vi "Process.vi"(8 "error in":errorcluster, 11 "Example Instrument UI":refnum<class "Instrument UI.Element2.lvclass">) -> (0 "error out":errorcluster, 3 "Example Instrument UI out":refnum<class "Instrument UI.Element2.lvclass">)   [LabVIEW 2019, in "Instrument UI.Element2.lvclass"]
doc: "---------------------------------------------------------------\nJKI State Machine Objects™\nhttp://jki.net/state-machine-objects/\nCopyright (C) 2005-2015, JKI <info@jki.net>\nALL RIGHTS RESERVEDJKI State Machine Objects (SMO) 1.0.0.5\nJKI - JKI\nCopyright (c) 2016, JKI"
uses:
  Instrument UI.Element2.lvclass
  C:/Program Files (x86)/National Instruments/LabVIEW 2019/vi.lib/JKI/JKI SMO/SMO/SMO.lvclass
  C:/Program Files (x86)/National Instruments/LabVIEW 2019/user.lib/LevyLab/Instrument Framework/SMOs/Instrument UI/Instrument UI.lvclass
  C:/Program Files (x86)/National Instruments/LabVIEW 2019/vi.lib/JKI/JKI SMO/SMO.UI/SMO.UI.lvclass
  Instrument.Element2/Typedefs/Instrument.Element2.getAll--Cluster.ctl
  Instrument.Element2/Instrument.Element2.lvclass
  C:/Program Files (x86)/National Instruments/LabVIEW 2019/user.lib/LevyLab/Instrument Framework/SMOs/Instrument/Instrument.lvclass
  Instrument UI.Element2.UI--Cluster.ctl
  Instrument.Element2/Typedefs/Instrument.Element2.Configuration--Cluster.ctl
  <userlib>/LevyLab/Instrument Framework/SMOs/Configuration/Configuration.lvclass
  <userlib>/LevyLab/Instrument Framework/SMOs/Instrument UI/Instrument UI.lvclass/Instrument UI.ctl
  <vilib>/JKI/JKI SMO/SMO/SMO.lvclass/SMO.ctl
  <userlib>/LevyLab/Instrument Framework/SMOs/Instrument/Instrument.lvclass/Instrument.ctl
  Instrument.Element2/Typedefs/Instrument.Element2.Commands--Enum.ctl
  614f1787-3484-4d72-b522-1f8c221dac07.vi
  812ceb25-51ea-4cc0-8aed-c299bc5e652a.vi
  5dc85c1f-8602-43a5-ace5-4d37edcece4b.vi
  199af190-1d6b-4486-8e47-a22270e27068.vi
  f46c0021-6761-4a3c-b250-c526aef0bf8a.vi
  a4c54d18-a951-4ce5-af52-fd32c219282c.vi
  508c6769-fd37-4c88-a163-d37e27e9b26a.vi
  d8b42418-d514-49a9-b82b-7ff31fc1bdce.vi
  4297835d-582f-4ffd-a274-1469935fba4e.vi
  9a5046e7-2a90-4c6a-9e24-f775917da756.vi
  064e3a37-d4cf-416d-9c97-81a00de9d50c.vi
  <vilib>/JKI/JKI SMO/SMO/Private/ReftoDVR--SMO.vi
  614f1787-3484-4d72-b522-1f8c221dac07.vi/8473158c-15b0-4583-96f4-657a0a8663aa.vi
  812ceb25-51ea-4cc0-8aed-c299bc5e652a.vi/b3a63406-e986-4e92-9c3b-61d3b3f5e845.vi
  <userlib>/LevyLab/Instrument Framework/SMOs/Instrument/API/Send and Receive.vi
  5dc85c1f-8602-43a5-ace5-4d37edcece4b.vi/c2ea8b73-9e98-4876-b80f-f9b76f4e6007.vi
  199af190-1d6b-4486-8e47-a22270e27068.vi/885cf8f8-053e-4c02-a193-c26a5fc5fd2e.vi
  f46c0021-6761-4a3c-b250-c526aef0bf8a.vi/d39bdf40-357d-4b84-b6e1-0fa9a47eb352.vi
  a4c54d18-a951-4ce5-af52-fd32c219282c.vi/e6982fbf-8c58-4b4e-8d6c-ef964828a5ea.vi
  508c6769-fd37-4c88-a163-d37e27e9b26a.vi/c2cd9c33-c0f3-4ea8-8363-db61e99eb68f.vi
  d8b42418-d514-49a9-b82b-7ff31fc1bdce.vi/7908e09d-14a4-4f19-b705-d41f2a7bdd7f.vi
  4297835d-582f-4ffd-a274-1469935fba4e.vi/ae23a806-acf6-4b68-963a-90a4cd4bdf43.vi
  9a5046e7-2a90-4c6a-9e24-f775917da756.vi/aa9366ea-5b79-4087-9b0d-90153f2fc7d9.vi
  064e3a37-d4cf-416d-9c97-81a00de9d50c.vi/3b377202-371f-4596-b702-b3c926413c9d.vi
  614f1787-3484-4d72-b522-1f8c221dac07.vi/8473158c-15b0-4583-96f4-657a0a8663aa.vi/a83233ea-3f32-419c-97c8-4d037e5cf615.vi
  812ceb25-51ea-4cc0-8aed-c299bc5e652a.vi/b3a63406-e986-4e92-9c3b-61d3b3f5e845.vi/6ae25757-18c0-4edf-8ec6-5ee7498e42bc.vi
  812ceb25-51ea-4cc0-8aed-c299bc5e652a.vi/b3a63406-e986-4e92-9c3b-61d3b3f5e845.vi/ba664fe4-fbf7-4d22-b628-f2801aca82a6.vi
  5dc85c1f-8602-43a5-ace5-4d37edcece4b.vi/c2ea8b73-9e98-4876-b80f-f9b76f4e6007.vi/1e7106c2-e63d-4954-be79-ade3d086157d.vi
  5dc85c1f-8602-43a5-ace5-4d37edcece4b.vi/c2ea8b73-9e98-4876-b80f-f9b76f4e6007.vi/5273b4ab-85e4-43b8-966e-2f27bfd0b167.vi
  199af190-1d6b-4486-8e47-a22270e27068.vi/885cf8f8-053e-4c02-a193-c26a5fc5fd2e.vi/98bda066-dba2-44b6-a77b-658504ed82f7.vi
  199af190-1d6b-4486-8e47-a22270e27068.vi/885cf8f8-053e-4c02-a193-c26a5fc5fd2e.vi/85f2e53d-7bfa-45b4-936c-816543ada8b5.vi
  f46c0021-6761-4a3c-b250-c526aef0bf8a.vi/d39bdf40-357d-4b84-b6e1-0fa9a47eb352.vi/fff4bc55-b81b-4902-9052-ccea61a7805f.vi
  f46c0021-6761-4a3c-b250-c526aef0bf8a.vi/d39bdf40-357d-4b84-b6e1-0fa9a47eb352.vi/8e797443-0d66-4240-84e1-5cfe0d1267f8.vi
  a4c54d18-a951-4ce5-af52-fd32c219282c.vi/e6982fbf-8c58-4b4e-8d6c-ef964828a5ea.vi/d1cd9f94-2750-44a9-b431-0a9c43ba5784.vi
  a4c54d18-a951-4ce5-af52-fd32c219282c.vi/e6982fbf-8c58-4b4e-8d6c-ef964828a5ea.vi/7fd59099-3350-4db8-8eec-f4e447bc4942.vi
  508c6769-fd37-4c88-a163-d37e27e9b26a.vi/c2cd9c33-c0f3-4ea8-8363-db61e99eb68f.vi/e3fa67e6-a539-4712-b44b-6125dcbb05d4.vi
  508c6769-fd37-4c88-a163-d37e27e9b26a.vi/c2cd9c33-c0f3-4ea8-8363-db61e99eb68f.vi/023fab8a-09d3-4eb7-ae02-fd4ece76aac4.vi
  d8b42418-d514-49a9-b82b-7ff31fc1bdce.vi/7908e09d-14a4-4f19-b705-d41f2a7bdd7f.vi/0e3d71bf-4189-4105-849b-527ecaac9cd6.vi
  d8b42418-d514-49a9-b82b-7ff31fc1bdce.vi/7908e09d-14a4-4f19-b705-d41f2a7bdd7f.vi/ea41837a-8cf8-405a-9125-7913f32814bd.vi
  4297835d-582f-4ffd-a274-1469935fba4e.vi/ae23a806-acf6-4b68-963a-90a4cd4bdf43.vi/9f397512-bf51-4fde-81a7-7db753787438.vi
  4297835d-582f-4ffd-a274-1469935fba4e.vi/ae23a806-acf6-4b68-963a-90a4cd4bdf43.vi/dd848b74-03c7-4bc3-8844-5b3e47300b5e.vi
  9a5046e7-2a90-4c6a-9e24-f775917da756.vi/aa9366ea-5b79-4087-9b0d-90153f2fc7d9.vi/42cffef1-50ff-4d5f-87eb-c31c2d9921ce.vi
  9a5046e7-2a90-4c6a-9e24-f775917da756.vi/aa9366ea-5b79-4087-9b0d-90153f2fc7d9.vi/f97c7ae1-12fc-4289-a497-f57069b3a3b7.vi
  064e3a37-d4cf-416d-9c97-81a00de9d50c.vi/3b377202-371f-4596-b702-b3c926413c9d.vi/9a630cf9-65e1-4d6a-a759-0b0e5b61d144.vi
  614f1787-3484-4d72-b522-1f8c221dac07.vi/8473158c-15b0-4583-96f4-657a0a8663aa.vi/a83233ea-3f32-419c-97c8-4d037e5cf615.vi/7e6555d9-0260-4203-9cda-f5732bbb5bfe.vi
  614f1787-3484-4d72-b522-1f8c221dac07.vi/8473158c-15b0-4583-96f4-657a0a8663aa.vi/a83233ea-3f32-419c-97c8-4d037e5cf615.vi/e950cb7d-6eaf-4b82-ab84-ba08af2cf0bb.vi
  064e3a37-d4cf-416d-9c97-81a00de9d50c.vi/3b377202-371f-4596-b702-b3c926413c9d.vi/9a630cf9-65e1-4d6a-a759-0b0e5b61d144.vi/9bda2bf0-22a8-471b-9ceb-dc726eacd9f3.vi
  064e3a37-d4cf-416d-9c97-81a00de9d50c.vi/3b377202-371f-4596-b702-b3c926413c9d.vi/9a630cf9-65e1-4d6a-a759-0b0e5b61d144.vi/6c670a7e-983d-46cc-b509-b9c25e863d4c.vi
  <userlib>/LevyLab/Instrument Framework/SMOs/Instrument/API/Enum to String.vi
  <userlib>/LevyLab/Instrument Framework/SMOs/RemoteControl/API/Send and Receive.vi
  <vilib>/Utility/Data Type/Get Type Information.vi
  <vilib>/JDP Science/JSONtext/JSON text to Variant.vi
  <userlib>/LevyLab/Instrument Framework/SMOs/Instrument/Instrument.lvclass
  <vilib>/JDP Science/JSONtext/LVClass Serializer/JSONtext LVClass Serializer.lvclass
  <userlib>/LevyLab/Instrument Framework/SMOs/Instrument UI/Instrument UI.lvclass
  <vilib>/JKI/JKI SMO/SMO/SMO.lvclass
  <vilib>/JKI/JKI SMO/SMO.UI/SMO.UI.lvclass
panel:
  out "Diode Current (A)":dbl
  out "Temperature (C)":dbl
  out "Error":bool
  out "Shutter":bool
  out "Laser":bool
  in  "Send Custom":bool
  in  "CustomString":string
  in  "Clear Errors":bool
  in  "Update Time":bool
  in  "Clear Shutdown":bool
  in  "Clear Wakeup":bool
  in  "Set Shutdown":bool
  in  "Shutdown Time":timestamp
  in  "Stop":bool
  in  "Start":bool
  out "Pump Power (W)":dbl
  in  "Wakeup Time":timestamp
  out "Status":string
  in  "Parameter 2":string
  out "Numeric":u32
  in  "Set Wakeup":bool
  in  "Parameter":dbl
  in  "Exit":bool
  # "Element 2 Monitor"
  # "SMO UI Template"
  # "For instructions on how to use the JKI State Machine Objects, examples and video tutorials, visit:\nhttp://jki.net/state-machine-objects/\n\nJKI State Machine Objects™\nhttp://jki.net/state-machine-objects/\nCopyright (C) 2005-2015, JKI <info@jki.net>\nALL RIGHTS RESERVED"
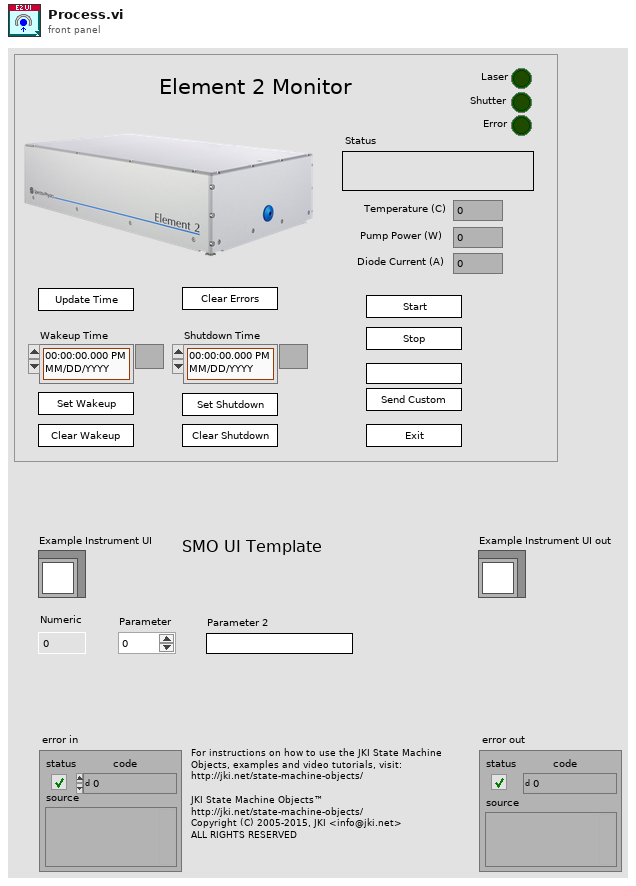
[diagram p1: front panel]
types:
  T1 = enum32{"invalid app kind", "Development System", "Run Time System", "Student Edition", "Embedded LabVIEW", "Evaluation", "Custom"}
  T2 = enum32{"Invalid", "Standard", "Closed", "Hidden", "Minimized", "Maximized"}
  T3 = typedef "Instrument.Element2.lvclass/Instrument.Element2.Commands--Enum.ctl" = enum16{"Start", "Stop", "Set Wakeup", "Clear Wakeup", "Set Shutdown", "Clear Shutdown", "Clear Errors", "Update Time", "Send Custom"}
  T4 = typedef "Instrument.Element2.lvclass/Instrument.Element2.Configuration--Cluster.ctl" = cluster{"Example Setting 1":dbl}
  T5 = typedef "Instrument.Element2.lvclass/Instrument.Element2.getAll--Cluster.ctl" = cluster{"Pump Power":dbl, "Laser Status":string, "Startup/Shutdown Status":string, "Diode Current Set":dbl, "Diode Current Actual":dbl, "Temp: Pump Chassis":dbl, "Temp: Pump PCB":dbl, "Temp: Pump Tower":dbl, "Temp: Pump Diodes":dbl, "Temp: Control Unit":dbl, "Temp: Laser Head Pos 1":dbl, "Temp: Laser Head Pos 2":dbl}
  T6 = typedef "Instrument UI.Element2.lvclass/Instrument UI.Element2.UI--Cluster.ctl" = cluster{"Parameter":dbl, "Parameter 2":string}
  T7 = cluster{"Core":cluster{"Current VI Reference":refnum<vi>, "Close Panel on Exit?":bool, "error":errorcluster}, "Instrument UI":refnum<class "Instrument UI.Element2.lvclass">, "Instrument":refnum<class "Instrument.Element2.lvclass">, "Configuration":refnum<class "Configuration.lvclass">, "Config Cluster":T4, "getAll":T5, "UI Cluster":T6}
  T8 = cluster{"Current VI Reference":refnum<vi>, "Close Panel on Exit?":bool, "error":errorcluster}
  T9 = typedef "SMO.lvclass/Protected Events.ctl" = cluster{"StopProcesses":refnum<user-event>, "AbortProcesses":refnum<user-event>, "Config Changed":refnum<user-event>, "Dependency":refnum<user-event>}
  T10 = typedef "Instrument.lvclass/PublicEvents--Cluster.ctl" = cluster{"MessageFromProcess":refnum<user-event>}
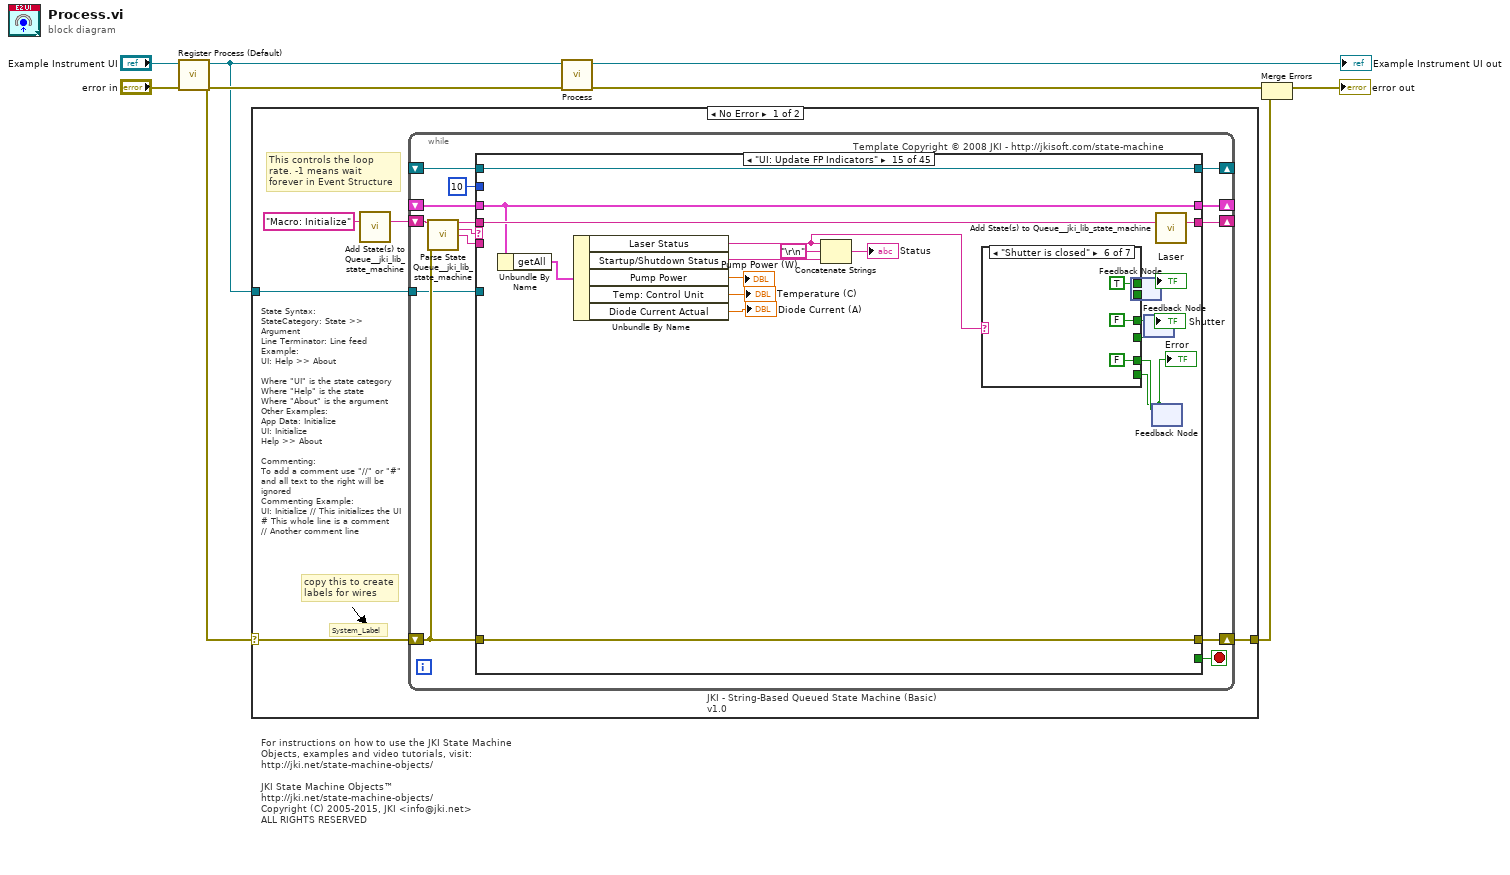
[diagram p0: block diagram]
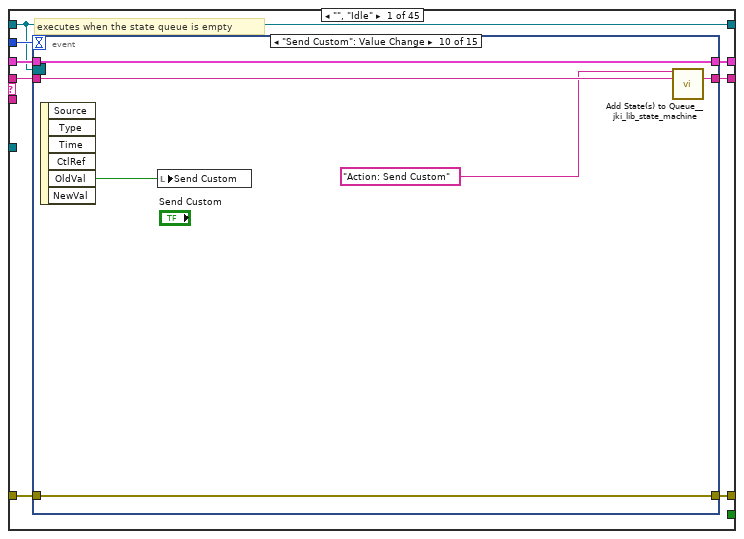
[diagram p2: hidden frame]
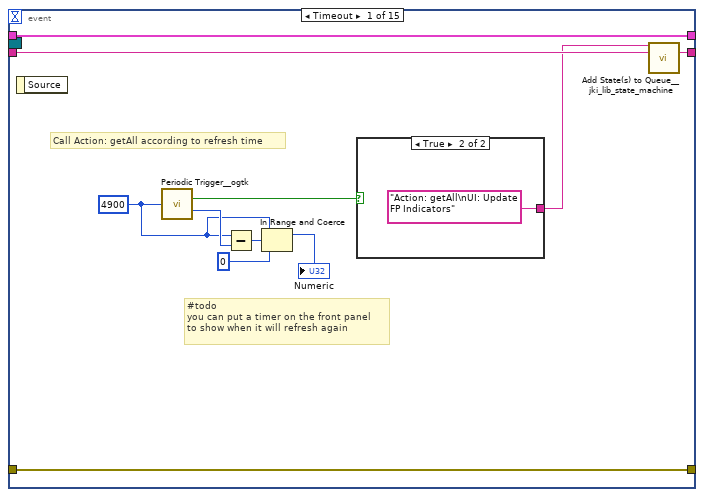
[diagram p3: hidden frame]
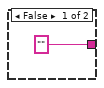
[diagram p4: hidden frame]
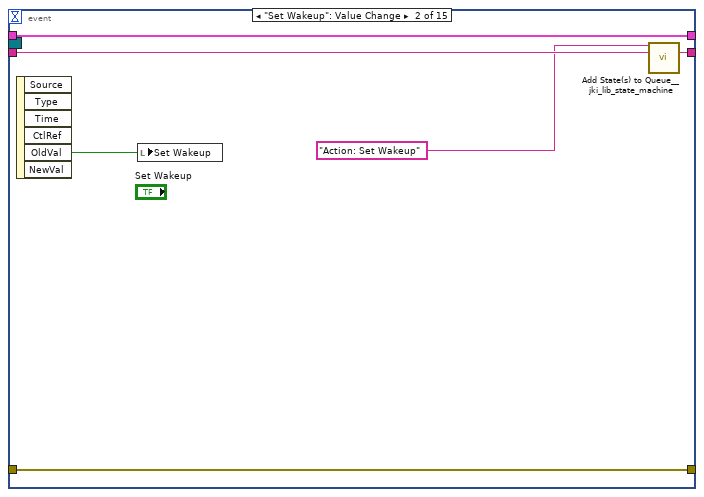
[diagram p5: hidden frame]
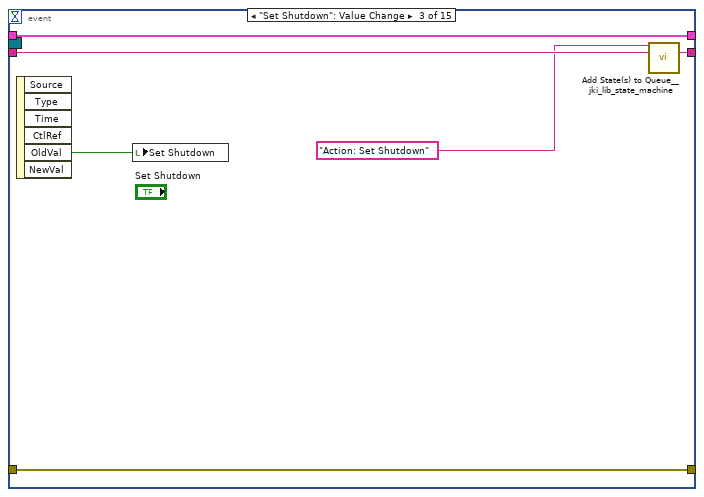
[diagram p6: hidden frame]
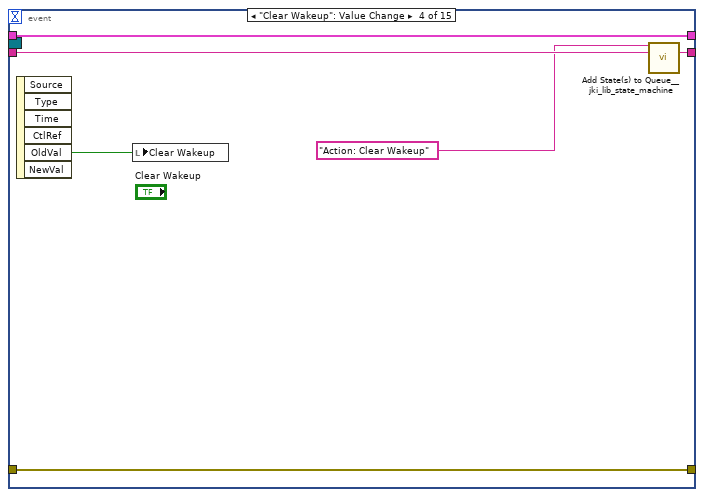
[diagram p7: hidden frame]
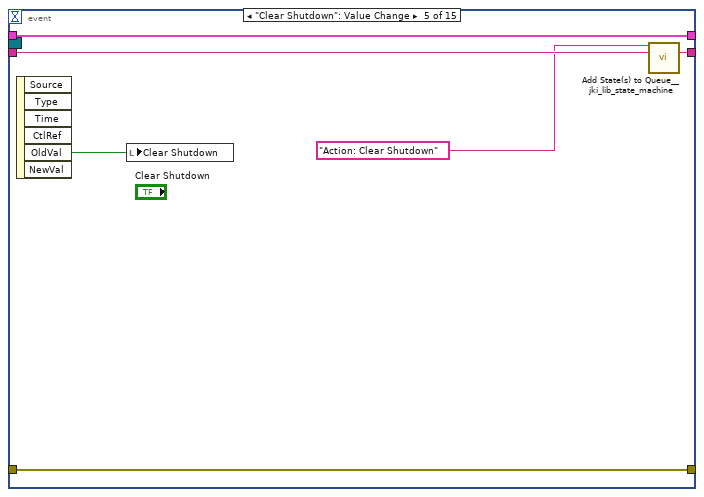
[diagram p8: hidden frame]
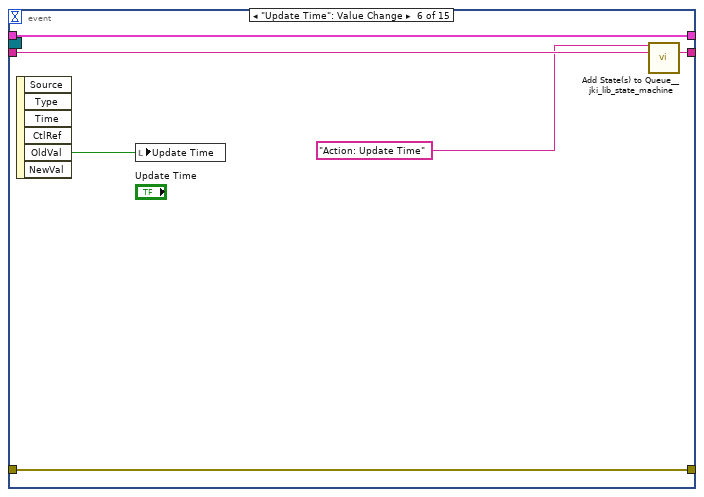
[diagram p9: hidden frame]
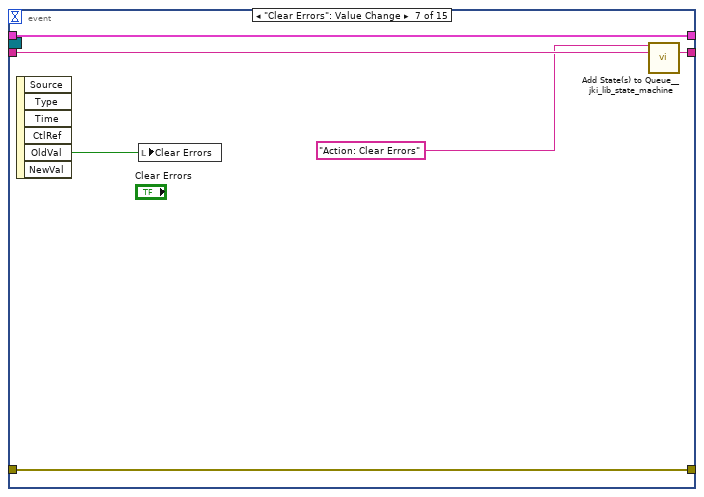
[diagram p10: hidden frame]
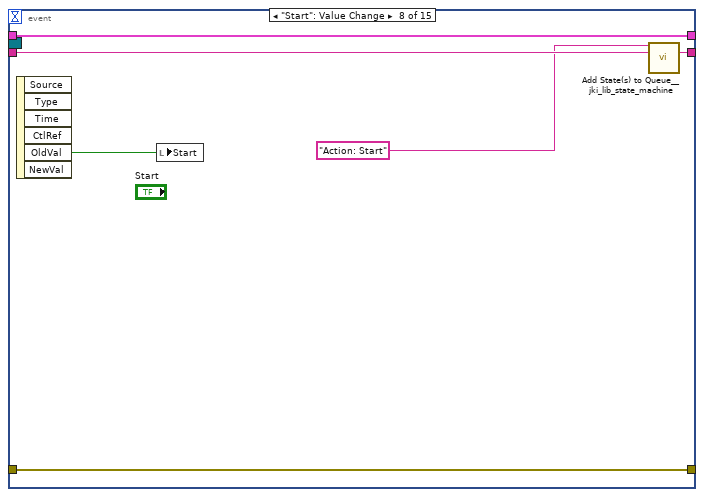
[diagram p11: hidden frame]
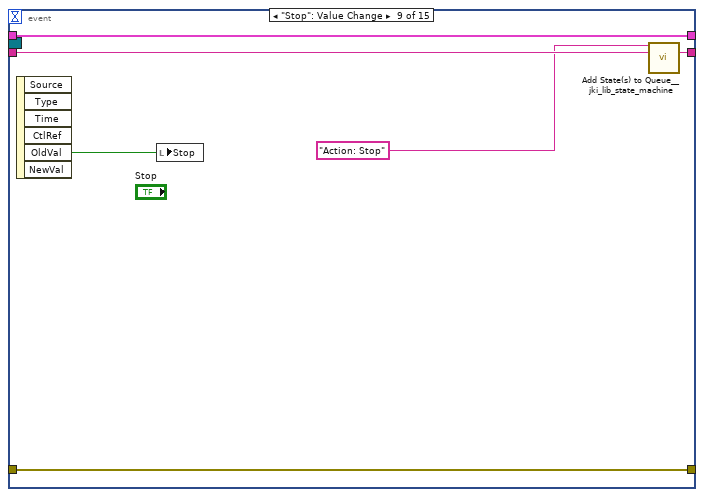
[diagram p12: hidden frame]
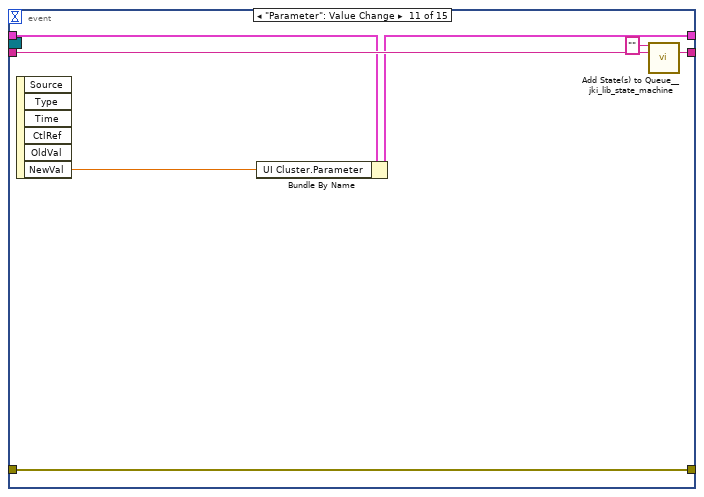
[diagram p13: hidden frame]
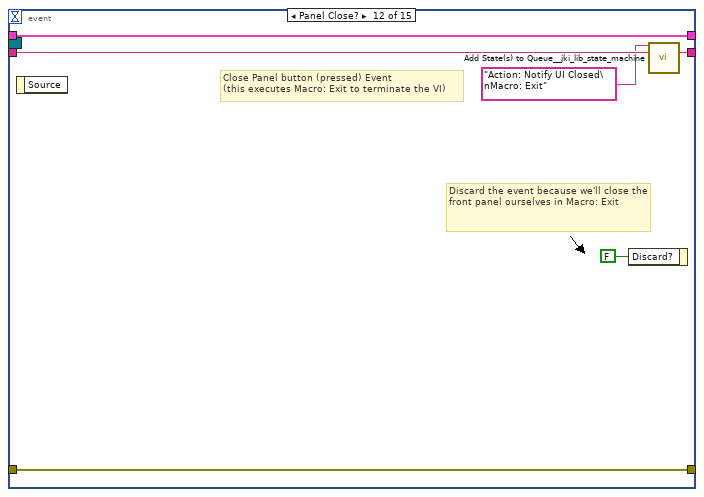
[diagram p14: hidden frame]
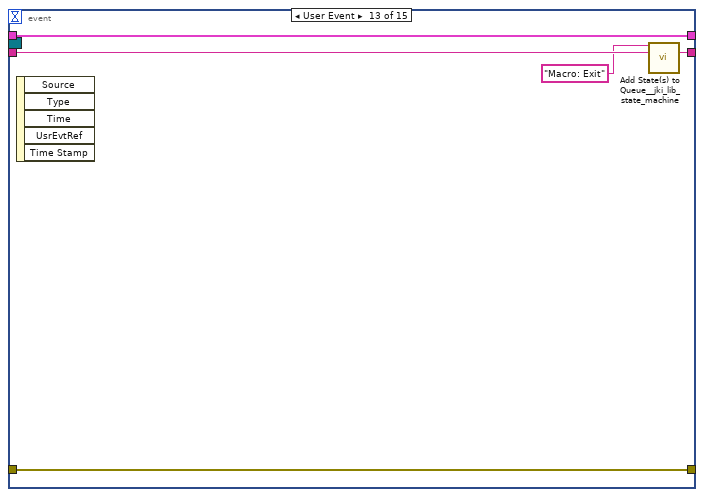
[diagram p15: hidden frame]
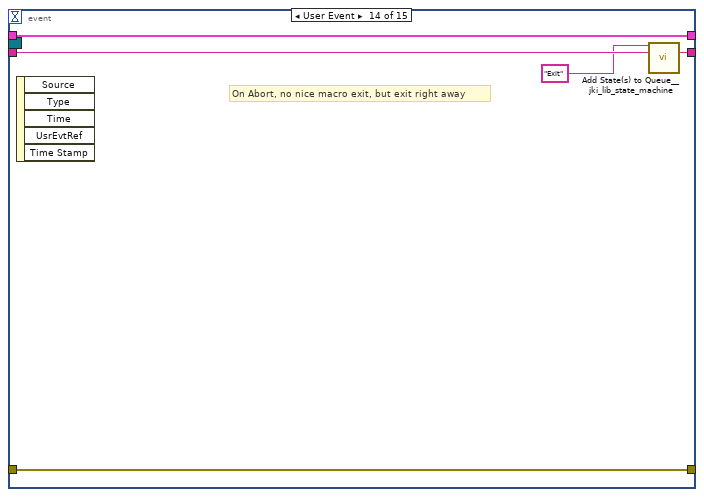
[diagram p16: hidden frame]
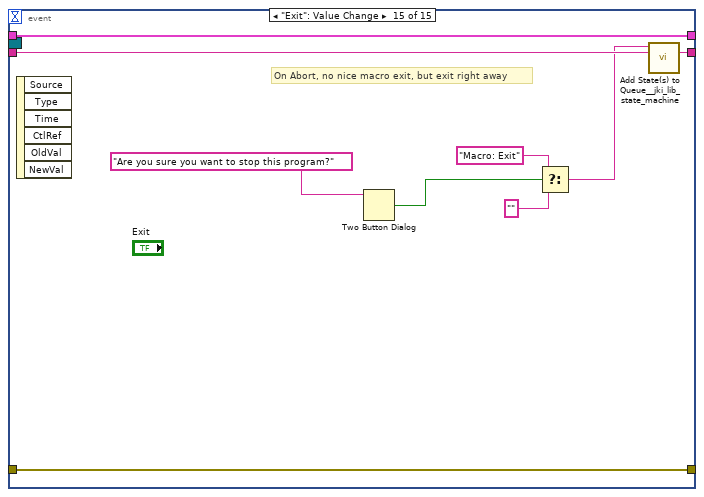
[diagram p17: hidden frame]
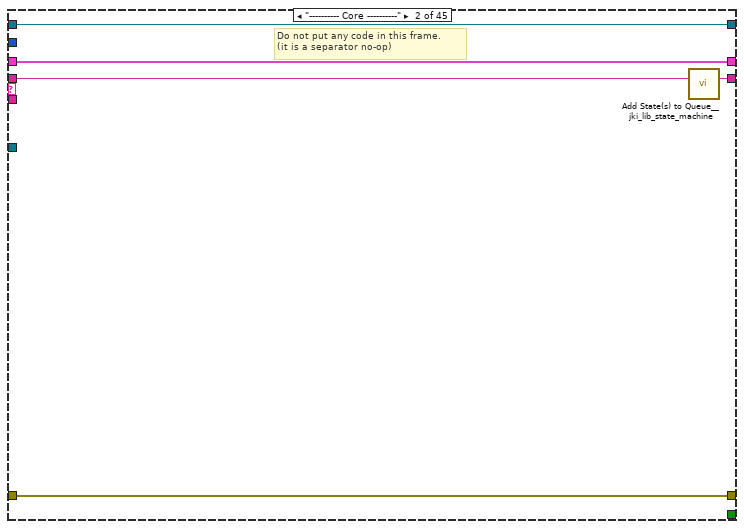
[diagram p18: hidden frame]
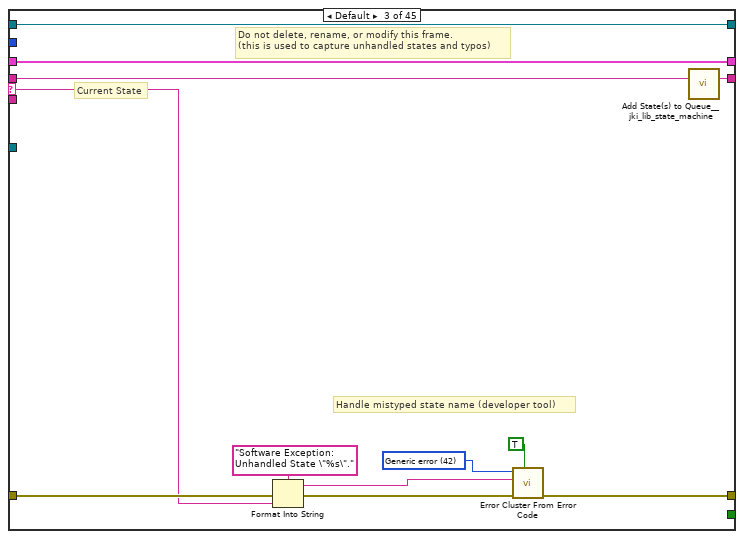
[diagram p19: hidden frame]
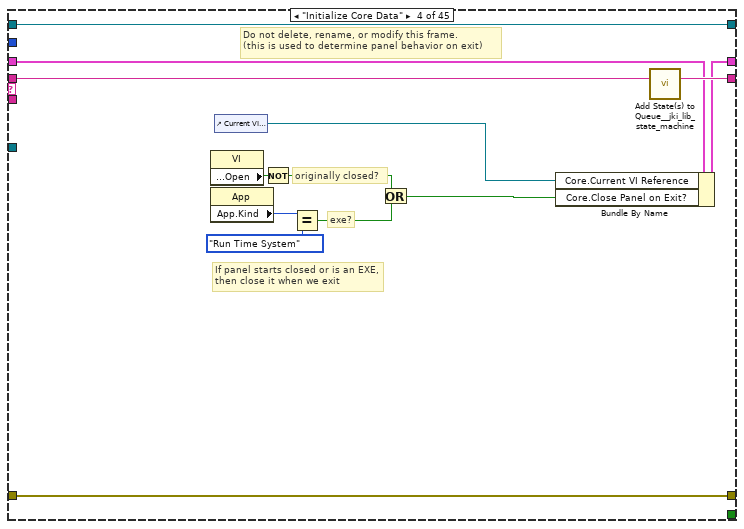
[diagram p20: hidden frame]
diagram:
  # "For instructions on how to use the JKI State Machine Objects, examples and video tutorials, visit:\nhttp://jki.net/state-machine-objects/\n\nJKI State Machine Objects™\nhttp://jki.net/state-machine-objects/\nCopyright (C) 2005-2015, JKI <info@jki.net>\nALL RIGHTS RESERVED"
  n1 = call <vilib>:"Register Process (Default).vi"("error in (no error)"="error in", "SMO"="Example Instrument UI") -> ("error out"=w5:errorcluster, "SelfRef"=w4:refnum<class "Instrument UI.Element2.lvclass">)  [unwired: 8 in]
  n2 = case shown="No Error" w5 {
    selector: w5 -> [w10 w603]
    tunnel: w4 -> [w11 _]
    tunnel: [w9 w603] -> w1
    frame No Error {
      # "State Syntax:\nStateCategory: State >> Argument\nLine Terminator: Line feed\nExample:\nUI: Help >> About\n\nWhere \"UI\" is the state category\nWhere \"Help\" is the state\nWhere \"About\" is the argument\nOther Examples:\nApp Data: Initialize\nUI: Initialize\nHelp >> About\n\nCommenting:\nTo add a comment use \"//\" or \"#\" and all text to the right will be ignored\nCommenting Example:\nUI: Initialize // This initializes the UI\n# This whole line is a comment\n// Another comment line"
      # "copy this to create labels for wires"
      # "This controls the loop rate. -1 means wait forever in Event Structure"
      # "System_Label"
      n3 = call <vilib>:"Add State(s) to Queue__jki_lib_state_machine.vi"("State(s) in (\"\")"="Macro: Initialize") -> ("States Out"=w13:string)  [unwired: 14 in]
      n4 = while "JKI - String-Based Queued State Machine (Basic) v1.0" {
        shift-right: [w20] -> _
        shift-left: _ -> [w19]
        shift-right: [w23] -> w9
        shift-left: w10 -> [w17]
        shift-right: [w22] -> _
        shift-left: w13 -> [w24]
        tunnel: w11 -> [w16]
        shift-right: [w15] -> _
        shift-left: _ -> [w14]
        stop <- w21 stop-if-true
        # "Template Copyright © 2008 JKI - http://jkisoft.com/state-machine"
        n5 = call <vilib>:"Parse State Queue__jki_lib_state_machine.vi"("State Queue"=w24, "Error In (no error)"=w17) -> ("Remaining States"=w26:string, "Current State"=w27:string, "Arguments"=w25:string)  [unwired: 11 in]
        n6 = case shown="\"UI: Update FP Indicators\"" w27 {
          selector: w27 -> [_ _ w141 _ _ _ _ _ _ _ _ _ _ _ _ _ _ _ _ _ _ _ _ _ _ _ _ _ _ _ _ _ _ _ _ _ _ _ _ _ _ _ _ _ _]
          tunnel: w26 -> [w35 w139 w145 w164 w178 w184 w189 w209 w217 w222 w229 w234 w241 w248 w267 w295 w311 w343 w352 w358 w364 w379 w384 w395 w402 w407 w420 w426 w431 w443 w451 w463 w470 w477 w489 w501 w513 w524 w535 w546 w557 w568 w579 w591 w602]
          tunnel: w25 -> [_ _ _ _ _ _ _ _ _ _ _ _ _ _ _ w289 w305 _ _ _ _ _ _ _ _ _ _ _ _ _ _ _ _ _ _ _ _ _ _ _ _ _ _ _ _]
          tunnel: w19 -> [w33 w136 w143 w155 w167 w180 w186 _ w213 w218 w223 w231 w239 w244 w262 w293 w307 w340 w348 w355 w361 w366 w381 w392 w397 w404 w418 w424 w428 w434 w448 w454 w466 w471 w481 w496 w508 w519 w530 w541 w552 w563 w574 w586 w594]
          tunnel: [w32 w137 w147 w161 w169 w179 w187 w191 w215 w220 w225 w232 w236 w246 w263 w290 w308 w341 w350 w356 w362 w377 w382 w386 w398 w405 w413 w421 w429 w438 w446 w455 w467 w472 w486 w492 w504 w515 w526 w537 w548 w559 w570 w582 w599] -> w23
          tunnel: w17 -> [w31 w137 w146 w161 w174 _ w187 w206 w215 w220 w226 w232 w237 w246 w263 w291 w309 w341 w350 w356 w362 w377 w382 w387 w399 w405 w415 w422 w429 w436 w444 w456 w467 w473 w482 w493 w505 w516 w527 w538 w549 w560 w571 w583 w595]
          tunnel: [w34 w138 w144 w163 w177 w183 w188 w208 w216 w221 w228 w233 w240 w247 w266 w294 w310 w342 w351 w357 w363 w378 w383 w394 w401 w406 w419 w425 w430 w442 w450 w462 w469 w476 w488 w500 w512 w523 w534 w545 w556 w567 w578 w590 w601] -> w22
          tunnel: [_ _ _ _ _ TRUE _ _ _ _ _ _ _ _ _ _ _ _ _ _ _ _ _ _ _ _ _ _ _ _ _ _ _ _ _ _ _ _ _ _ _ _ _ _ _] -> w21
          tunnel: [w30 w136 w143 w162 w166 w180 w186 w207 w212 w218 w223 w231 w239 w244 w262 w293 w307 w340 w348 w355 w361 w366 w381 w392 w397 w404 w418 w424 w428 w440 w448 w452 w465 w471 w483 w497 w509 w520 w531 w542 w553 w564 w575 w587 w596] -> w20
          tunnel: 10 ("Timeout") -> [w29 _ _ _ _ _ _ _ _ _ _ _ _ _ _ _ _ _ _ _ _ _ _ _ _ _ _ _ _ _ _ _ _ _ _ _ _ _ _ _ _ _ _ _ _]
          tunnel: w16 -> [_ _ _ _ _ _ _ w204 _ _ _ _ _ _ _ _ _ _ _ _ _ _ _ _ _ _ _ _ _ _ _ _ _ _ _ _ _ _ _ _ _ _ _ _ _]
          tunnel: [w28 w135 w140 w152 w176 w181 w185 w203 w214 w219 w224 w230 w238 w245 w265 w292 w304 w339 w349 w354 w360 w371 w380 w393 w400 w403 w417 w423 w427 w441 w449 w461 w468 w475 w487 w499 w511 w522 w533 w544 w555 w566 w577 w589 w600] -> w15
          tunnel: w14 -> [w28 w135 w140 w152 w176 w181 w185 w203 w214 w219 w224 w230 w238 w245 w265 w292 w304 w339 w349 w354 w360 w371 w380 w393 w400 w403 _ w423 w427 w441 w449 w461 w468 w475 w487 w499 w511 w522 w533 w544 w555 w566 w577 w589 w600]
          frame "", "Idle" {
            # "executes when the state queue is empty"
            n7 = event shown="[9] \"Send Custom\": Value Change" {
              selector: w28 -> [_ _ _ _ _ _ _ _ _ _ _ _ _ _ _]
              dyn-events: _ -> [_ _ _ _ _ _ _ _ _ _ _ _ _ _ _]
              timeout: w29 -> [_ _ _ _ _ _ _ _ _ _ _ _ _ _ _]
              tunnel: w35 -> [w46 w54 w60 w66 w72 w78 w84 w90 w96 w102 w109 w115 w120 w125 w134]
              tunnel: [w45 w53 w59 w65 w71 w77 w83 w89 w95 w101 w108 w114 w119 w124 w133] -> w34
              tunnel: w33 -> [w43 w51 w57 w63 w69 w75 w81 w87 w93 w99 w105 w111 w117 w122 w131]
              tunnel: [w44 w52 w58 w64 w70 w76 w82 w88 w94 w100 w107 w110 w118 w123 w132] -> w32
              tunnel: w31 -> [w44 w52 w58 w64 w70 w76 w82 w88 w94 w100 w107 w110 w118 w123 w132]
              tunnel: [w43 w51 w57 w63 w69 w75 w81 w87 w93 w99 w104 w111 w117 w122 w131] -> w30
              event Timeout {
                w37 = u32 4900 ("time (ms)")
                # "#todo\nyou can put a timer on the front panel\nto show when it will refresh again"
                # "Call Action: getAll according to refresh time"
                n8 = event-data() -> ()  [unwired: 1 in, 1 out]
                n9 = call <userlib>:"Periodic Trigger__ogtk.vi"("time (ms)"=w37) -> ("Triggered"=w41:bool, "timer value"=w40:u32)  [unwired: 12 in, 1 out]
                n10 = Subtract(x=w37, y=w40) -> (x-y=w39:u32)
                n11 = In Range and Coerce(upper limit=w37, x=w39, lower limit=u32 0) -> (coerced(x)=→"Numeric":u32)  [unwired: 1 out]
                n12 = case shown="True" w41 {
                  tunnel: ["" ("State(s) in Front (\"\")") "Action: getAll\nUI: Update FP Indicators" ("State(s) in Front (\"\")")] -> w42
                  frame False {
                  }
                  frame True {
                  }
                }
                n13 = call <vilib>:"Add State(s) to Queue__jki_lib_state_machine.vi"("State(s) in Front (\"\")"=w42, "State(s) in (\"\")"=w46) -> ("States Out"=w45:string)  [unwired: 13 in]
              }
              event "Set Wakeup": Value Change {
                n14 = event-data() -> ("OldVal"=w50:bool)  [unwired: 1 in, 5 out]
                n15 = local write "Set Wakeup"(w50) -> ()
                n16 = call <vilib>:"Add State(s) to Queue__jki_lib_state_machine.vi"("State(s) in Front (\"\")"="Action: Set Wakeup" ("State(s) in Front (\"\")"), "State(s) in (\"\")"=w54) -> ("States Out"=w53:string)  [unwired: 13 in]
              }
              event "Set Shutdown": Value Change {
                n17 = event-data() -> ("OldVal"=w56:bool)  [unwired: 1 in, 5 out]
                n18 = local write "Set Shutdown"(w56) -> ()
                n19 = call <vilib>:"Add State(s) to Queue__jki_lib_state_machine.vi"("State(s) in Front (\"\")"="Action: Set Shutdown" ("State(s) in Front (\"\")"), "State(s) in (\"\")"=w60) -> ("States Out"=w59:string)  [unwired: 13 in]
              }
              event "Clear Wakeup": Value Change {
                n20 = event-data() -> ("OldVal"=w62:bool)  [unwired: 1 in, 5 out]
                n21 = local write "Clear Wakeup"(w62) -> ()
                n22 = call <vilib>:"Add State(s) to Queue__jki_lib_state_machine.vi"("State(s) in Front (\"\")"="Action: Clear Wakeup" ("State(s) in Front (\"\")"), "State(s) in (\"\")"=w66) -> ("States Out"=w65:string)  [unwired: 13 in]
              }
              event "Clear Shutdown": Value Change {
                n23 = event-data() -> ("OldVal"=w68:bool)  [unwired: 1 in, 5 out]
                n24 = local write "Clear Shutdown"(w68) -> ()
                n25 = call <vilib>:"Add State(s) to Queue__jki_lib_state_machine.vi"("State(s) in Front (\"\")"="Action: Clear Shutdown" ("State(s) in Front (\"\")"), "State(s) in (\"\")"=w72) -> ("States Out"=w71:string)  [unwired: 13 in]
              }
              event "Update Time": Value Change {
                n26 = event-data() -> ("OldVal"=w74:bool)  [unwired: 1 in, 5 out]
                n27 = local write "Update Time"(w74) -> ()
                n28 = call <vilib>:"Add State(s) to Queue__jki_lib_state_machine.vi"("State(s) in Front (\"\")"="Action: Update Time" ("State(s) in Front (\"\")"), "State(s) in (\"\")"=w78) -> ("States Out"=w77:string)  [unwired: 13 in]
              }
              event "Clear Errors": Value Change {
                n29 = event-data() -> ("OldVal"=w80:bool)  [unwired: 1 in, 5 out]
                n30 = local write "Clear Errors"(w80) -> ()
                n31 = call <vilib>:"Add State(s) to Queue__jki_lib_state_machine.vi"("State(s) in Front (\"\")"="Action: Clear Errors" ("State(s) in Front (\"\")"), "State(s) in (\"\")"=w84) -> ("States Out"=w83:string)  [unwired: 13 in]
              }
              event "Start": Value Change {
                n32 = event-data() -> ("OldVal"=w86:bool)  [unwired: 1 in, 5 out]
                n33 = local write "Start"(w86) -> ()
                n34 = call <vilib>:"Add State(s) to Queue__jki_lib_state_machine.vi"("State(s) in Front (\"\")"="Action: Start" ("State(s) in Front (\"\")"), "State(s) in (\"\")"=w90) -> ("States Out"=w89:string)  [unwired: 13 in]
              }
              event "Stop": Value Change {
                n35 = event-data() -> ("OldVal"=w92:bool)  [unwired: 1 in, 5 out]
                n36 = local write "Stop"(w92) -> ()
                n37 = call <vilib>:"Add State(s) to Queue__jki_lib_state_machine.vi"("State(s) in Front (\"\")"="Action: Stop" ("State(s) in Front (\"\")"), "State(s) in (\"\")"=w96) -> ("States Out"=w95:string)  [unwired: 13 in]
              }
              event "Send Custom": Value Change {
                n38 = event-data() -> ("OldVal"=w98:bool)  [unwired: 1 in, 5 out]
                n39 = local write "Send Custom"(w98) -> ()
                n40 = call <vilib>:"Add State(s) to Queue__jki_lib_state_machine.vi"("State(s) in Front (\"\")"="Action: Send Custom" ("State(s) in Front (\"\")"), "State(s) in (\"\")"=w102) -> ("States Out"=w101:string)  [unwired: 13 in]
              }
              event "Parameter": Value Change {
                n41 = event-data() -> ("NewVal"=w106:dbl)  [unwired: 1 in, 5 out]
                n42 = Bundle By Name(cluster=w105, "UI Cluster.Parameter"=w106) -> (w104:T7)
                n43 = call <vilib>:"Add State(s) to Queue__jki_lib_state_machine.vi"("State(s) in Front (\"\")"="" ("State(s) in Front (\"\")"), "State(s) in (\"\")"=w109) -> ("States Out"=w108:string)  [unwired: 13 in]
              }
              event Panel Close? {
                # "Discard the event because we'll close the front panel ourselves in Macro: Exit"
                # "Close Panel button (pressed) Event\n(this executes Macro: Exit to terminate the VI)"
                n44 = event-data() -> ()  [unwired: 1 in, 1 out]
                n45 = event-data("Discard?"=FALSE) -> ()  [unwired: 1 in, 1 out]
                n46 = call <vilib>:"Add State(s) to Queue__jki_lib_state_machine.vi"("State(s) in Front (\"\")"="Action: Notify UI Closed\nMacro: Exit", "State(s) in (\"\")"=w115) -> ("States Out"=w114:string)  [unwired: 13 in]
              }
              event User Event {
                n47 = event-data() -> ()  [unwired: 1 in, 5 out]
                n48 = call <vilib>:"Add State(s) to Queue__jki_lib_state_machine.vi"("State(s) in Front (\"\")"="Macro: Exit", "State(s) in (\"\")"=w120) -> ("States Out"=w119:string)  [unwired: 13 in]
              }
              event User Event {
                # "On Abort, no nice macro exit, but exit right away"
                n49 = event-data() -> ()  [unwired: 1 in, 5 out]
                n50 = call <vilib>:"Add State(s) to Queue__jki_lib_state_machine.vi"("State(s) in Front (\"\")"="Exit", "State(s) in (\"\")"=w125) -> ("States Out"=w124:string)  [unwired: 13 in]
              }
              event "Exit": Value Change {
                # "On Abort, no nice macro exit, but exit right away"
                n51 = event-data() -> ()  [unwired: 1 in, 6 out]
                n52 = Two Button Dialog(message="Are you sure you want to stop this program?") -> (T button?=w130:bool)  [unwired: 2 in]
                n53 = Select(t="Macro: Exit", s=w130, f="") -> (s? t:f=w126:string)
                n54 = call <vilib>:"Add State(s) to Queue__jki_lib_state_machine.vi"("State(s) in Front (\"\")"=w126, "State(s) in (\"\")"=w134) -> ("States Out"=w133:string)  [unwired: 13 in]
              }
            }
          }
          frame "---------- Core ----------" {
            # "Do not put any code in this frame.\n(it is a separator no-op)"
            n55 = call <vilib>:"Add State(s) to Queue__jki_lib_state_machine.vi"("State(s) in (\"\")"=w139) -> ("States Out"=w138:string)  [unwired: 14 in]
          }
          frame Default {
            w150 = 42 items=["No error", "Argument error", "Memory is full", "Out of zone", "End of file", "File already open", "Generic file I/O error", "File not found", "File permission error", "Disk is full", "Duplicate path", "Too many files open", "System feature not enabled", "Resource file not found", "Cannot add resource", "Resource not found", "Image not found", "Image memory error", "Pen does not exist", "Config type invalid", "Config token not found", "Config parse error", "Config memory error", "Bad external code format", "Bad external code offset", "External code not present", "Null window", "Destroy window error", "Null menu", "Print aborted", "Bad print record", "Print driver error", "Windows error during printing", "Memory error during printing", "Print dialog error", "Generic print error", "Invalid device refnum", "Device not found", "Device parameter error", "Device unit error", "Cannot open device", "Device call aborted", "Generic error", "Cancelled by user", "Object ID too low", "Object ID too high", "Object not in heap", "Unknown heap", "Unknown object (invalid DefProc)", "Unknown object (DefProc not in table)", "Message out of range", "Invalid (null) method", "Unknown message", "Manager call not supported", "Bad address", "Network operation in progress", "Network operation timed out", "Connection is busy", "Network attribute not supported", "Network error", "Address in use", "System out of memory", "Connection aborted", "Connection refused", "Not connected", "Already connected", "Connection closed", "Initialization error (interapplication manager)", "Bad occurrence", "Wait on unbound occurrence handler", "Occurrence queue overflow", "Datalog type conflict", "Unused", "Unrecognized type (interapplication manager)", "Memory corrupt", "Failed to make temporary DLL", "Old CIN version", "Drag socket not found", "Failed to load drop-object", "Failed to register OLE object", "Failed to release OLE object", "Format specifier type mismatch", "Unknown format specifier", "Too few format specifiers", "Too many format specifiers", "Scan failed", "Newer CIN version", "Error converting to variant", "Runtime menu error", "Password tampered", "Variant attribute not found", "Incompatible variant data type", "Event data is not available", "Event Store is not present", "Occurrence is not found", "Event Queue is not created", "Event info is not available", "Refnum passed is NULL", "Error retrieving Class GUID", "Error retrieving CoClass GUID", "Error retrieving TypeLib GUID.", "Bad built application magic bytes.", "Specific driver is different from the specific driver associated with the Logical Name.", "There is no session opened to the class driver.", "Max Error", "MAX - Error with config objects", "MAX - Error loading configuration", "MAX - Group not supported"]
            # "Current State"
            # "Do not delete, rename, or modify this frame.\n(this is used to capture unhandled states and typos)"
            # "Handle mistyped state name (developer tool)"
            n56 = Format Into String(format string="Software Exception: Unhandled State \"%s\"." ("message"), error in=w146, w141) -> (resulting string=w149:string, error out=w148:errorcluster)  [unwired: 1 in]
            n57 = call <vilib>:"Error Cluster From Error Code.vi"("show call chain? (False)"=TRUE, "error in (no error)"=w148, "error message (\"\")"=w149, "error code (0)"=w150) -> ("error out"=w147:errorcluster)  [unwired: 5 in]
            n58 = call <vilib>:"Add State(s) to Queue__jki_lib_state_machine.vi"("State(s) in (\"\")"=w145) -> ("States Out"=w144:string)  [unwired: 14 in]
          }
          frame "Initialize Core Data" {
            # "Do not delete, rename, or modify this frame.\n(this is used to determine panel behavior on exit)"
            # "originally closed?"
            # "exe?"
            # "If panel starts closed or is an EXE, then close it when we exit"
            n59 = property class="VI"() -> ("Front Panel.Open"=w160:bool)  [unwired: 2 in, 2 out]
            n60 = property class="App"() -> ("App.Kind"=w159:T1)  [unwired: 2 in, 2 out]
            n61 = control-ref of="Current VI Reference"() -> (w153:refnum<vi>)
            n62 = Not(x=w160) -> (.not. x?=w157:bool)
            n63 = Equal?(x=w159, y=T1."Run Time System" ("Application:Kind")) -> (x = y?=w156:bool)
            n64 = Or(x=w157, y=w156) -> (x .or. y?=w154:bool)
            n65 = Bundle By Name(cluster=w155, "Core.Current VI Reference"=w153, "Core.Close Panel on Exit?"=w154) -> (w162:T7)
            n66 = call <vilib>:"Add State(s) to Queue__jki_lib_state_machine.vi"("State(s) in (\"\")"=w164) -> ("States Out"=w163:string)  [unwired: 14 in]
          }
          frame "Error Handler" {
            w169 = errorcluster {"status"=FALSE, "code"=0, "source"=""}  # No error
            # "Overwrite this method to handle errors and pass to parent if not handled. Parent will fire a public event if the error is not handled up the chain of classes."
            # "Handle any errors here.\nYou can also output any states to clean-up after errors occur"
            n67 = Unbundle By Name(w167) -> ("Instrument UI"=w175:refnum<class "Instrument UI.Element2.lvclass">)
            n68 = call-dynamic "Handle Error.vi"("Stop on Unhandled Error (T)"=FALSE, "error in"=w174, "SMO"=w175) -> ("handling error"=w170:errorcluster, "Unhandled error"=w168:errorcluster)  [unwired: 6 in, 1 out]
            n69 = Bundle By Name(cluster=w167, "Core.error"=w168) -> (w166:T7)
            n70 = Select(t="Exit", s=w170, f="") -> (s? t:f=w171:string)
            n71 = call <vilib>:"Add State(s) to Queue__jki_lib_state_machine.vi"("State(s) in Front (\"\")"=w171, "State(s) in (\"\")"=w178) -> ("States Out"=w177:string)  [unwired: 13 in]
          }
          frame "Exit" {
            # "Do not put any code in this frame.\n(No errors that occur here will be handled.)"
            n72 = Unbundle By Name(w180) -> ("Core.error"=w179:errorcluster)
            n73 = call <vilib>:"Add State(s) to Queue__jki_lib_state_machine.vi"("State(s) in (\"\")"=w184) -> ("States Out"=w183:string)  [unwired: 14 in]
          }
          frame "---------- Data ----------" {
            # "Do not put any code in this frame.\n(It is a separator no-op. You can make a copy of this frame to create a new Data frame)"
            n74 = call <vilib>:"Add State(s) to Queue__jki_lib_state_machine.vi"("State(s) in (\"\")"=w189) -> ("States Out"=w188:string)  [unwired: 14 in]
          }
          frame "Data: Initialize" {
            w190 = refnum<class "Configuration.lvclass"> refnum  # Configuration
            w193 = T4 {"Example Setting 1"=0.0}  # Config Cluster
            w195 = T6 {"Parameter"=0.0, "Parameter 2"=""}  # UI Cluster
            w197 = refnum<class "Instrument.Element2.lvclass"> refnum  # Instrument
            w201 = T5 {"Pump Power"=0.0, "Laser Status"="", "Startup/Shutdown Status"="", "Diode Current Set"=0.0, "Diode Current Actual"=0.0, "Temp: Pump Chassis"=0.0, "Temp: Pump PCB"=0.0, "Temp: Pump Tower"=0.0, "Temp: Pump Diodes"=0.0, "Temp: Control Unit"=0.0, "Temp: Laser Head Pos 1"=0.0, "Temp: Laser Head Pos 2"=0.0}  # getAll
            w202 = T8 {"Current VI Reference"=refnum, "Close Panel on Exit?"=FALSE, "error"={"status"=FALSE, "code"=0, "source"=""}}  # Core
            w205 = refnum<class "Instrument UI.Element2.lvclass"> refnum  # Self Reference
            # "typedef from Child Instrument"
            # "Cluster of UI\ninformation you\nwant to save/load"
            # "Child Instrument"
            # "typedef from Child Instrument"
            # "do not delete - used by framework"
            # "Data names and types of shift register data are defined by this bundle."
            # "Initialize the shift-register data, here.\n(data names are defined by what you wire into the bundle function)"
            n75 = Variant To Data(error in=w206, type=w205, Variant=w204) -> (data=w199:refnum<class "Instrument UI.Element2.lvclass">, error out=w200:errorcluster)
            n76 = call <userlib>:"Read Instrument.vi"("error in (no error)"=w200, "Instrument UI in"=w199) -> ("error out"=w194:errorcluster, "Instrument"=w196:refnum<class "Instrument.lvclass">, "Instrument UI"=w198:refnum<class "Instrument UI.Element2.lvclass">)  [unwired: 7 in]
            n77 = To More Specific Class(target class=w197, reference=w196, error in=w194) -> (specific class reference=w192:refnum<class "Instrument.Element2.lvclass">, error out=w191:errorcluster)
            n78 = Bundle("Core"=w202, "Instrument UI"=w198, "Instrument"=w192, "Configuration"=w190, "Config Cluster"=w193, "getAll"=w201, "UI Cluster"=w195) -> (w207:T7)  [unwired: 1 in]
            n79 = call <vilib>:"Add State(s) to Queue__jki_lib_state_machine.vi"("State(s) in (\"\")"=w209) -> ("States Out"=w208:string)  [unwired: 14 in]
          }
          frame "Data: Set UI Cluster" {
            # "Do not put any code in this frame.\n(It is a separator no-op. You can make a copy of this frame to create a new Data frame)"
            n80 = Bundle By Name(cluster=w213, "UI Cluster.Parameter"="Parameter", "UI Cluster.Parameter 2"="Parameter 2") -> (w212:T7)
            n81 = call <vilib>:"Add State(s) to Queue__jki_lib_state_machine.vi"("State(s) in (\"\")"=w217) -> ("States Out"=w216:string)  [unwired: 14 in]
          }
          frame "Data: Set Config Cluster" {
            # "Do not put any code in this frame.\n(It is a separator no-op. You can make a copy of this frame to create a new Data frame)"
            n82 = call <vilib>:"Add State(s) to Queue__jki_lib_state_machine.vi"("State(s) in (\"\")"=w222) -> ("States Out"=w221:string)  [unwired: 14 in]
          }
          frame "Data: Cleanup" {
            # "Cleanup any data and references, here.\n(this is called automatically, by the Macro: Exit)"
            n83 = Unbundle By Name(w223) -> ("Core.Current VI Reference"=w227:refnum<vi>)
            n84 = Close Reference(reference=w227, error in (no error)=w226) -> (error out=w225:errorcluster)
            n85 = call <vilib>:"Add State(s) to Queue__jki_lib_state_machine.vi"("State(s) in (\"\")"=w229) -> ("States Out"=w228:string)  [unwired: 14 in]
          }
          frame "---------- UI ----------" {
            # "Do not put any code in this frame.\n(It is a separator no-op. You can make a copy of this frame to create a new UI frame)"
            n86 = call <vilib>:"Add State(s) to Queue__jki_lib_state_machine.vi"("State(s) in (\"\")"=w234) -> ("States Out"=w233:string)  [unwired: 14 in]
          }
          frame "UI: Initialize" {
            # "size window to decoration box on front panel"
            # "Initialize the User Interface, here.\n(this is called automatically, by the Macro: Init)"
            n87 = invoke on="Exit" class="Bool (strict)" method="Reinit To Default"() -> ()  [unwired: 3 in, 3 out]
            n88 = call <userlib>:"Fit VI window to Largest Dec__ogtk.vi"("error in (no error)"=w237, "border spacing (2 px)"=0) -> ("error out"=w236:errorcluster)  [unwired: 4 in, 1 out]
            n89 = call <vilib>:"Add State(s) to Queue__jki_lib_state_machine.vi"("State(s) in (\"\")"=w241) -> ("States Out"=w240:string)  [unwired: 14 in]
          }
          frame "UI: Update FP Controls" {
            # "Do not put any code in this frame.\n(It is a separator no-op. You can make a copy of this frame to create a new UI frame)"
            n90 = Unbundle By Name(w244) -> ("UI Cluster.Parameter"=w242:dbl, "UI Cluster.Parameter 2"=w243:string)
            n91 = local write "Parameter 2"(w243) -> ()
            n92 = local write "Parameter"(w242) -> ()
            n93 = call <vilib>:"Add State(s) to Queue__jki_lib_state_machine.vi"("State(s) in (\"\")"=w248) -> ("States Out"=w247:string)  [unwired: 14 in]
          }
          frame "UI: Update FP Indicators" {
            n94 = Unbundle By Name(w262) -> ("getAll"=w264:T5)
            n95 = Unbundle By Name(w264) -> ("Laser Status"=w257:string, "Startup/Shutdown Status"=w261:string, "Pump Power"=→"Pump Power (W)":dbl, "Temp: Control Unit"=→"Temperature (C)":dbl, "Diode Current Actual"=→"Diode Current (A)":dbl)
            n96 = Concatenate Strings(w257, "\r\n", w261) -> (→"Status":string)
            n97 = feedback #1() -> (w251:bool)  [unwired: 1 in]
            "Laser" <- w251
            n98 = feedback #2() -> (w249:bool)  [unwired: 1 in]
            "Shutter" <- w249
            n99 = feedback #3() -> (w255:bool)  [unwired: 1 in]
            "Error" <- w255
            n100 = case shown="\"Shutter is closed\"" w257 {
              tunnel: [w269 TRUE ("Laser") FALSE ("Laser") FALSE ("Laser") TRUE ("Laser") TRUE ("Laser") FALSE ("Laser")] -> w252
              tunnel: [w270 FALSE ("Error") TRUE ("Error") TRUE ("Error") FALSE ("Error") FALSE ("Error") FALSE ("Error")] -> w256
              tunnel: [w268 w271 FALSE ("Shutter") FALSE ("Shutter") TRUE ("Shutter") FALSE ("Shutter") FALSE ("Shutter")] -> w250
              tunnel: w255 -> [w270 _ _ _ _ _ _]
              tunnel: w251 -> [w269 _ _ _ _ _ _]
              tunnel: w249 -> [w268 w271 _ _ _ _ _]
              frame "False", Default {
              }
              frame "LASER is RUNNING" {
              }
              frame "Maintenance" {
              }
              frame "1 Error detected !" {
              }
              frame "Shutter is open" {
              }
              frame "Shutter is closed" {
              }
              frame "STANDBY" {
              }
            }
            n101 = feedback-in #1(w252) -> ()
            n102 = feedback-in #2(w250) -> ()
            n103 = feedback-in #3(w256) -> ()
            n104 = call <vilib>:"Add State(s) to Queue__jki_lib_state_machine.vi"("State(s) in (\"\")"=w267) -> ("States Out"=w266:string)  [unwired: 14 in]
          }
          frame "UI: Cursor Set" {
            # "Argument"
            # "Initialize the User Interface, here.\n(this is called automatically, by the Macro: Init)"
            n105 = disable-structure shown="Default" {
              disable-tunnel: w291 -> [w296 w299]
              disable-tunnel: [w296 w298] -> w290
              disable-tunnel: w289 -> [_ w297]
              frame condition #0 {
              }
              frame condition #1 (active) {
                n106 = case shown="\"Busy\"" w297 {
                  tunnel: w299 -> [w301 w303]
                  tunnel: [w300 w302] -> w298
                  frame "Idle", Default {
                    n107 = call <vilib>:"Unset Busy.vi"("error in (no error)"=w301) -> ("error out"=w300:errorcluster)  [unwired: 10 in]
                  }
                  frame "Busy" {
                    n108 = call <vilib>:"Set Busy.vi"("error in (no error)"=w303) -> ("error out"=w302:errorcluster)  [unwired: 9 in, 1 out]
                  }
                }
              }
            }
            n109 = call <vilib>:"Add State(s) to Queue__jki_lib_state_machine.vi"("State(s) in (\"\")"=w295) -> ("States Out"=w294:string)  [unwired: 14 in]
          }
          frame "UI: Front Panel State" {
            # "Argument"
            # "Set Front Panel Open or Closed\n(Usage: \"UI: Front Panel State >> Open|Close\")"
            n110 = Unbundle By Name(w307) -> ("Core.Current VI Reference"=w306:refnum<vi>)
            n111 = disable-structure shown="Default" {
              disable-tunnel: w309 -> [w315 w338]
              disable-tunnel: [w314 w338] -> w308
              disable-tunnel: w306 -> [w313 _]
              disable-tunnel: w305 -> [w312 _]
              frame condition #0 (active) {
                n112 = case shown="\"Close\"" w312 {
                  tunnel: w315 -> [w319 w332]
                  tunnel: [w321 w333] -> w314
                  tunnel: w313 -> [w320 w330]
                  frame "Open", Default {
                    n113 = property class="VI"(reference=w320, error in=w319) -> (reference out=w317:refnum<vi>, error out=w318:errorcluster, "FP.State"=w316:T2)
                    n114 = case shown="\"Closed\"" w316 {
                      tunnel: [w324 w327] -> w321
                      tunnel: w318 -> [w323 w327]
                      tunnel: w317 -> [w322 _]
                      frame "Closed" {
                        n115 = invoke class="VI" method="FP.Open"(reference=w322, error in=w323, "Activate"=TRUE, "State"=T2."Standard") -> (error out=w324:errorcluster)  [unwired: 1 in, 4 out]
                      }
                      frame Default {
                      }
                    }
                  }
                  frame "Close" {
                    n116 = property class="VI"(reference=w330, error in=w332) -> (reference out=w329:refnum<vi>, error out=w331:errorcluster, "FP.State"=w328:T2)
                    n117 = case shown="Default" w328 {
                      tunnel: [w334 w337] -> w333
                      tunnel: w331 -> [w334 w336]
                      tunnel: w329 -> [_ w335]
                      frame "Invalid", "Closed" {
                      }
                      frame Default {
                        n118 = invoke class="VI" method="FP.Close"(reference=w335, error in=w336) -> (error out=w337:errorcluster)  [unwired: 1 in, 2 out]
                      }
                    }
                  }
                }
              }
              frame condition #1 {
              }
            }
            n119 = call <vilib>:"Add State(s) to Queue__jki_lib_state_machine.vi"("State(s) in (\"\")"=w311) -> ("States Out"=w310:string)  [unwired: 14 in]
          }
          frame "---------- Macro ----------" {
            # "Do not put any code in this frame.\n(It is a separator no-op. You can make a copy of this frame to create a new Macro frame)"
            n120 = call <vilib>:"Add State(s) to Queue__jki_lib_state_machine.vi"("State(s) in (\"\")"=w343) -> ("States Out"=w342:string)  [unwired: 14 in]
          }
          frame "Macro: Initialize" {
            w346 = "UI: Initialize\nMacro: Read UI Config\n//UI: Front Panel State >> Open"  # UI: Initialize Macro: Read UI Config //UI: Front Panel State >> Open
            # "Initialization Macro\n(This is called once, when the VI starts)"
            n121 = call <vilib>:"Add State(s) to Queue__jki_lib_state_machine.vi"("State(s) in Front (\"\")"="Data: Initialize\nInitialize Core Data\nEvents: Register", "State(s) in (\"\")"="Process: Sync", "State(s) at Back (\"\")"=w346) -> ("States Out"=w345:string)  [unwired: 12 in]
            n122 = call <vilib>:"Add State(s) to Queue__jki_lib_state_machine.vi"("State(s) in Front (\"\")"=w345, "State(s) in (\"\")"=w352) -> ("States Out"=w351:string)  [unwired: 13 in]
          }
          frame "Macro: Read UI Config" {
            # "Do not put any code in this frame.\n(It is a separator no-op. You can make a copy of this frame to create a new Macro frame)"
            n123 = call <vilib>:"Add State(s) to Queue__jki_lib_state_machine.vi"("State(s) in Front (\"\")"="Configuration: Initialize\nConfiguration: Read UI Config File\nUI: Update FP Controls" ("State(s) in Front (\"\")"), "State(s) in (\"\")"=w358) -> ("States Out"=w357:string)  [unwired: 13 in]
          }
          frame "Macro: Write UI Config" {
            # "Do not put any code in this frame.\n(It is a separator no-op. You can make a copy of this frame to create a new Macro frame)"
            n124 = call <vilib>:"Add State(s) to Queue__jki_lib_state_machine.vi"("State(s) in Front (\"\")"="Data: Set UI Cluster\nConfiguration: Write UI Config File" ("State(s) in Front (\"\")"), "State(s) in (\"\")"=w364) -> ("States Out"=w363:string)  [unwired: 13 in]
          }
          frame "Macro: Exit" {
            # "Exit Macro\n(This is called once, when the VI exits)"
            n125 = Unbundle By Name(w366) -> ("Core.Close Panel on Exit?"=w376:bool)
            n126 = Select(t="UI: Front Panel State >> Close", s=w376, f="") -> (s? t:f=w373:string)
            n127 = call <vilib>:"Add State(s) to Queue__jki_lib_state_machine.vi"("State(s) in Front (\"\")"="Data: Cleanup\nEvents: Unregister\nProcess: Self Terminate", "State(s) in (\"\")"="Process: Sync", "State(s) at Back (\"\")"="Exit") -> ("States Out"=w368:string)  [unwired: 12 in]
            n128 = call <vilib>:"Add State(s) to Queue__jki_lib_state_machine.vi"("State(s) in Front (\"\")"="Macro: Write UI Config", "State(s) in (\"\")"=w373, "State(s) at Back (\"\")"=w368) -> ("States Out"=w372:string)  [unwired: 12 in]
            n129 = call <vilib>:"Add State(s) to Queue__jki_lib_state_machine.vi"("State(s) in Front (\"\")"=w372, "State(s) in (\"\")"=w379) -> ("States Out"=w378:string)  [unwired: 13 in]
          }
          frame "---------- Process ----------" {
            # "Template Separator\n(You can make a copy of, or modify, this frame)"
            n130 = call <vilib>:"Add State(s) to Queue__jki_lib_state_machine.vi"("State(s) in (\"\")"=w384) -> ("States Out"=w383:string)  [unwired: 14 in]
          }
          frame "Process: Sync" {
            n131 = Unbundle By Name(w392) -> ("Instrument UI"=w388:refnum<class "Instrument UI.Element2.lvclass">)
            n132 = call <vilib>:"WaitOnProcessSync.vi"("error in (no error)"=w387, "SMO"=w388) -> ("error out"=w386:errorcluster, "Don't run?"=w391:bool)  [unwired: 7 in, 1 out]
            n133 = Select(t="Data: Cleanup\nEvents: Unregister\nExit", s=w391, f="") -> (s? t:f=w385:string)
            n134 = call <vilib>:"Add State(s) to Queue__jki_lib_state_machine.vi"("State(s) in Front (\"\")"=w385, "State(s) in (\"\")"=w395) -> ("States Out"=w394:string)  [unwired: 13 in]
          }
          frame "Process: Self Terminate" {
            n135 = Unbundle By Name(w397) -> ("Instrument UI"=w396:refnum<class "Instrument UI.Element2.lvclass">)
            n136 = call <vilib>:"SelfTerminate.vi"("error in (no error)"=w399, "SMO in"=w396) -> ("error out"=w398:errorcluster)  [unwired: 8 in, 1 out]
            n137 = call <vilib>:"Add State(s) to Queue__jki_lib_state_machine.vi"("State(s) in (\"\")"=w402) -> ("States Out"=w401:string)  [unwired: 14 in]
          }
          frame "---------- Events ----------" {
            # "Template Separator\n(You can make a copy of, or modify, this frame)"
            n138 = call <vilib>:"Add State(s) to Queue__jki_lib_state_machine.vi"("State(s) in (\"\")"=w407) -> ("States Out"=w406:string)  [unwired: 14 in]
          }
          frame "Events: Register" {
            # "Expand to add\nmore events"
            # "Base Class Protected Events"
            n139 = Unbundle By Name(w418) -> ("Instrument UI"=w409:refnum<class "Instrument UI.Element2.lvclass">, "Instrument"=w408:refnum<class "Instrument.Element2.lvclass">)
            n140 = call <vilib>:"GetProtectedEvents.vi"("SMO"=w409) -> ("error out"=w412:errorcluster, "SMO Protected Events"=w416:T9)  [unwired: 8 in, 1 out]
            n141 = call <userlib>:"Instrument.GetPublicEvents.vi"("Instrument"=w408) -> ("error out"=w410:errorcluster, "Instrument Public Events"=w411:T10)  [unwired: 8 in, 1 out]
            n142 = register-events(w416, w411) -> (reference out=w417:refnum<event-registration>, error out=w414:errorcluster)  [unwired: 2 in]
            n143 = Merge Errors(w410, w415, w414, w412) -> (w413:errorcluster)
            n144 = call <vilib>:"Add State(s) to Queue__jki_lib_state_machine.vi"("State(s) in (\"\")"=w420) -> ("States Out"=w419:string)  [unwired: 14 in]
          }
          frame "Events: Unregister" {
            n145 = Unregister For Events(event registration refnum=w423, error in=w422) -> (error out=w421:errorcluster)
            n146 = call <vilib>:"Add State(s) to Queue__jki_lib_state_machine.vi"("State(s) in (\"\")"=w426) -> ("States Out"=w425:string)  [unwired: 14 in]
          }
          frame "---------- Configuration ----------" {
            # "Do not put any code in this frame.\n(It is a separator no-op. You can make a copy of this frame to create a new UI frame)"
            n147 = call <vilib>:"Add State(s) to Queue__jki_lib_state_machine.vi"("State(s) in (\"\")"=w431) -> ("States Out"=w430:string)  [unwired: 14 in]
          }
          frame "Configuration: Initialize" {
            # "Do not put any code in this frame.\n(It is a separator no-op. You can make a copy of this frame to create a new UI frame)"
            n148 = Unbundle By Name(w434) -> ("Configuration"=w432:refnum<class "Configuration.lvclass">, "Instrument"=w433:refnum<class "Instrument.Element2.lvclass">)
            n149 = call <vilib>:"GetName.vi"("error in (no error)"=w436, "SMO"=w433) -> ("error out"=w435:errorcluster, "Name"=w437:string)  [unwired: 6 in, 2 out]
            n150 = call <userlib>:"Default Path.vi"("error in (no error)"=w435, "Folder Name"=w437, "Configuration in"=w432) -> ("error out"=w438:errorcluster, "Configuration out"=w439:refnum<class "Configuration.lvclass">)  [unwired: 7 in]
            n151 = Bundle By Name(cluster=w434, "Configuration"=w439) -> (w440:T7)
            n152 = call <vilib>:"Add State(s) to Queue__jki_lib_state_machine.vi"("State(s) in (\"\")"=w443) -> ("States Out"=w442:string)  [unwired: 14 in]
          }
          frame "Configuration: Write UI Config File" {
            # "Do not put any code in this frame.\n(It is a separator no-op. You can make a copy of this frame to create a new Data frame)"
            n153 = Unbundle By Name(w448) -> ("Configuration"=w445:refnum<class "Configuration.lvclass">, "UI Cluster"=w447:T6)
            n154 = call <userlib>:"Write Configuration.vi"("error in (no error)"=w444, "Variant"=w447, "Configuration in"=w445) -> ("error out"=w446:errorcluster)  [unwired: 7 in, 1 out]
            n155 = call <vilib>:"Add State(s) to Queue__jki_lib_state_machine.vi"("State(s) in (\"\")"=w451) -> ("States Out"=w450:string)  [unwired: 14 in]
          }
          frame "Configuration: Read UI Config File" {
            # "Do not put any code in this frame.\n(It is a separator no-op. You can make a copy of this frame to create a new UI frame)"
            n156 = Unbundle By Name(w454) -> ("UI Cluster"=w457:T6, "Configuration"=w460:refnum<class "Configuration.lvclass">)
            n157 = call <userlib>:"Read Configuration.vi"("INI Fomatted Cluster Type"=w457, "error in (no error)"=w456, "Configuration in"=w460) -> ("error out"=w459:errorcluster, "Configuration"=w458:variant)  [unwired: 6 in, 1 out]
            n158 = Variant To Data(error in=w459, type=w457, Variant=w458) -> (data=w453:T6, error out=w455:errorcluster)
            n159 = Bundle By Name(cluster=w454, "UI Cluster"=w453) -> (w452:T7)
            n160 = call <vilib>:"Add State(s) to Queue__jki_lib_state_machine.vi"("State(s) in (\"\")"=w463) -> ("States Out"=w462:string)  [unwired: 14 in]
          }
          frame "---------- Action ----------" {
            n161 = Unbundle By Name(w466) -> ("Instrument UI"=w464:refnum<class "Instrument UI.Element2.lvclass">)
            n162 = Bundle By Name(cluster=w466, "Instrument UI"=w464) -> (w465:T7)
            n163 = call <vilib>:"Add State(s) to Queue__jki_lib_state_machine.vi"("State(s) in (\"\")"=w470) -> ("States Out"=w469:string)  [unwired: 14 in]
          }
          frame "Action: Notify UI Closed" {
            # "Notify that the UI has been closed"
            n164 = Unbundle By Name(w471) -> ("Instrument UI"=w474:refnum<class "Instrument UI.Element2.lvclass">)
            n165 = call <vilib>:"Hide.vi"("error in (no error)"=w473, "SMO.UI"=w474) -> ("error out"=w472:errorcluster)  [unwired: 8 in, 1 out]
            n166 = call <vilib>:"Add State(s) to Queue__jki_lib_state_machine.vi"("State(s) in (\"\")"=w477) -> ("States Out"=w476:string)  [unwired: 14 in]
          }
          frame "Action: getAll" {
            n167 = Unbundle By Name(w481) -> ("getAll"=w479:T5, "Instrument"=w484:refnum<class "Instrument.Element2.lvclass">)
            n168 = call "GET ALL.vim"("type"=w479, "error in (no error)"=w482, "Instrument in"=w484) -> ("error out"=w486:errorcluster, "getAll"=w478:T5, "Instrument out"=w480:refnum<class "Instrument.Element2.lvclass">)  [unwired: 6 in]
            n169 = Bundle By Name(cluster=w481, "Instrument"=w480, "getAll"=w478) -> (w483:T7)
            n170 = call <vilib>:"Add State(s) to Queue__jki_lib_state_machine.vi"("State(s) in Front (\"\")"="" ("State(s) in Front (\"\")"), "State(s) in (\"\")"=w489) -> ("States Out"=w488:string)  [unwired: 13 in]
          }
          frame "Action: Set Wakeup" {
            n171 = Unbundle By Name(w496) -> ("Instrument"=w495:refnum<class "Instrument.Element2.lvclass">)
            n172 = call "Remote Client.vim"("error in (no error)"=w493, "params"="Wakeup Time", "method"=Instrument.Element2.Commands--Enum."Set Wakeup" ("Commands"), "Instrument in"=w495) -> ("error out"=w492:errorcluster, "Instrument out"=w494:refnum<class "Instrument.Element2.lvclass">)  [unwired: 4 in, 2 out]
            n173 = Bundle By Name(cluster=w496, "Instrument"=w494) -> (w497:T7)
            n174 = call <vilib>:"Add State(s) to Queue__jki_lib_state_machine.vi"("State(s) in Front (\"\")"="" ("State(s) in Front (\"\")"), "State(s) in (\"\")"=w501) -> ("States Out"=w500:string)  [unwired: 13 in]
          }
          frame "Action: Set Shutdown" {
            n175 = Unbundle By Name(w508) -> ("Instrument"=w507:refnum<class "Instrument.Element2.lvclass">)
            n176 = call "Remote Client.vim"("error in (no error)"=w505, "params"="Shutdown Time", "method"=Instrument.Element2.Commands--Enum."Set Shutdown" ("Commands"), "Instrument in"=w507) -> ("error out"=w504:errorcluster, "Instrument out"=w506:refnum<class "Instrument.Element2.lvclass">)  [unwired: 4 in, 2 out]
            n177 = Bundle By Name(cluster=w508, "Instrument"=w506) -> (w509:T7)
            n178 = call <vilib>:"Add State(s) to Queue__jki_lib_state_machine.vi"("State(s) in Front (\"\")"="" ("State(s) in Front (\"\")"), "State(s) in (\"\")"=w513) -> ("States Out"=w512:string)  [unwired: 13 in]
          }
          frame "Action: Start" {
            n179 = Unbundle By Name(w519) -> ("Instrument"=w518:refnum<class "Instrument.Element2.lvclass">)
            n180 = call "Remote Client.vim"("error in (no error)"=w516, "method"=Instrument.Element2.Commands--Enum."Start" ("Commands"), "Instrument in"=w518) -> ("error out"=w515:errorcluster, "Instrument out"=w517:refnum<class "Instrument.Element2.lvclass">)  [unwired: 5 in, 2 out]
            n181 = Bundle By Name(cluster=w519, "Instrument"=w517) -> (w520:T7)
            n182 = call <vilib>:"Add State(s) to Queue__jki_lib_state_machine.vi"("State(s) in Front (\"\")"="" ("State(s) in Front (\"\")"), "State(s) in (\"\")"=w524) -> ("States Out"=w523:string)  [unwired: 13 in]
          }
          frame "Action: Stop" {
            n183 = Unbundle By Name(w530) -> ("Instrument"=w529:refnum<class "Instrument.Element2.lvclass">)
            n184 = call "Remote Client.vim"("error in (no error)"=w527, "method"=Instrument.Element2.Commands--Enum."Stop" ("Commands"), "Instrument in"=w529) -> ("error out"=w526:errorcluster, "Instrument out"=w528:refnum<class "Instrument.Element2.lvclass">)  [unwired: 5 in, 2 out]
            n185 = Bundle By Name(cluster=w530, "Instrument"=w528) -> (w531:T7)
            n186 = call <vilib>:"Add State(s) to Queue__jki_lib_state_machine.vi"("State(s) in Front (\"\")"="" ("State(s) in Front (\"\")"), "State(s) in (\"\")"=w535) -> ("States Out"=w534:string)  [unwired: 13 in]
          }
          frame "Action: Clear Wakeup" {
            n187 = Unbundle By Name(w541) -> ("Instrument"=w540:refnum<class "Instrument.Element2.lvclass">)
            n188 = call "Remote Client.vim"("error in (no error)"=w538, "method"=Instrument.Element2.Commands--Enum."Clear Wakeup" ("Commands"), "Instrument in"=w540) -> ("error out"=w537:errorcluster, "Instrument out"=w539:refnum<class "Instrument.Element2.lvclass">)  [unwired: 5 in, 2 out]
            n189 = Bundle By Name(cluster=w541, "Instrument"=w539) -> (w542:T7)
            n190 = call <vilib>:"Add State(s) to Queue__jki_lib_state_machine.vi"("State(s) in Front (\"\")"="" ("State(s) in Front (\"\")"), "State(s) in (\"\")"=w546) -> ("States Out"=w545:string)  [unwired: 13 in]
          }
          frame "Action: Clear Shutdown" {
            n191 = Unbundle By Name(w552) -> ("Instrument"=w551:refnum<class "Instrument.Element2.lvclass">)
            n192 = call "Remote Client.vim"("error in (no error)"=w549, "method"=Instrument.Element2.Commands--Enum."Clear Shutdown" ("Commands"), "Instrument in"=w551) -> ("error out"=w548:errorcluster, "Instrument out"=w550:refnum<class "Instrument.Element2.lvclass">)  [unwired: 5 in, 2 out]
            n193 = Bundle By Name(cluster=w552, "Instrument"=w550) -> (w553:T7)
            n194 = call <vilib>:"Add State(s) to Queue__jki_lib_state_machine.vi"("State(s) in Front (\"\")"="" ("State(s) in Front (\"\")"), "State(s) in (\"\")"=w557) -> ("States Out"=w556:string)  [unwired: 13 in]
          }
          frame "Action: Update Time" {
            n195 = Unbundle By Name(w563) -> ("Instrument"=w562:refnum<class "Instrument.Element2.lvclass">)
            n196 = call "Remote Client.vim"("error in (no error)"=w560, "method"=Instrument.Element2.Commands--Enum."Update Time" ("Commands"), "Instrument in"=w562) -> ("error out"=w559:errorcluster, "Instrument out"=w561:refnum<class "Instrument.Element2.lvclass">)  [unwired: 5 in, 2 out]
            n197 = Bundle By Name(cluster=w563, "Instrument"=w561) -> (w564:T7)
            n198 = call <vilib>:"Add State(s) to Queue__jki_lib_state_machine.vi"("State(s) in Front (\"\")"="" ("State(s) in Front (\"\")"), "State(s) in (\"\")"=w568) -> ("States Out"=w567:string)  [unwired: 13 in]
          }
          frame "Action: Clear Errors" {
            n199 = Unbundle By Name(w574) -> ("Instrument"=w573:refnum<class "Instrument.Element2.lvclass">)
            n200 = call "Remote Client.vim"("error in (no error)"=w571, "method"=Instrument.Element2.Commands--Enum."Clear Errors" ("Commands"), "Instrument in"=w573) -> ("error out"=w570:errorcluster, "Instrument out"=w572:refnum<class "Instrument.Element2.lvclass">)  [unwired: 5 in, 2 out]
            n201 = Bundle By Name(cluster=w574, "Instrument"=w572) -> (w575:T7)
            n202 = call <vilib>:"Add State(s) to Queue__jki_lib_state_machine.vi"("State(s) in Front (\"\")"="" ("State(s) in Front (\"\")"), "State(s) in (\"\")"=w579) -> ("States Out"=w578:string)  [unwired: 13 in]
          }
          frame "Action: Send Custom" {
            n203 = Unbundle By Name(w586) -> ("Instrument"=w585:refnum<class "Instrument.Element2.lvclass">)
            n204 = call "Remote Client.vim"("error in (no error)"=w583, "params"="CustomString", "method"=Instrument.Element2.Commands--Enum."Send Custom" ("Commands"), "Instrument in"=w585) -> ("error out"=w582:errorcluster, "Instrument out"=w584:refnum<class "Instrument.Element2.lvclass">)  [unwired: 4 in, 2 out]
            n205 = Bundle By Name(cluster=w586, "Instrument"=w584) -> (w587:T7)
            n206 = call <vilib>:"Add State(s) to Queue__jki_lib_state_machine.vi"("State(s) in Front (\"\")"="" ("State(s) in Front (\"\")"), "State(s) in (\"\")"=w591) -> ("States Out"=w590:string)  [unwired: 13 in]
          }
          frame "Action: setConfiguration" {
            n207 = Unbundle By Name(w594) -> ("Instrument"=w597:refnum<class "Instrument.Element2.lvclass">, "Config Cluster"=w592:T4)
            n208 = call "SET CONFIG.vim"("error in (no error)"=w595, "Configuration"=w592, "Instrument in"=w597) -> ("error out"=w599:errorcluster, "Instrument out"=w593:refnum<class "Instrument.Element2.lvclass">)  [unwired: 7 in]
            n209 = Bundle By Name(cluster=w594, "Instrument"=w593) -> (w596:T7)
            n210 = call <vilib>:"Add State(s) to Queue__jki_lib_state_machine.vi"("State(s) in Front (\"\")"="" ("State(s) in Front (\"\")"), "State(s) in (\"\")"=w602) -> ("States Out"=w601:string)  [unwired: 13 in]
          }
        }
      }
    }
    frame Error {
    }
  }
  n211 = call-parent "Process.vi"("error in"=w5, "Instrument UI in"=w4) -> ("error out"=w2:errorcluster, "Instrument UI out"=→"Example Instrument UI out":refnum<class "Instrument UI.Element2.lvclass">)  [unwired: 8 in]
  n212 = Merge Errors(w2, w1) -> (→"error out":errorcluster)
